vi "Stage 3.6 Placing GUI into subVIs.vi"() -> ()   [LabVIEW 2020]
panel:
  out "Process Error":errorcluster
  out "error out":errorcluster
  out "error out Hardware":errorcluster
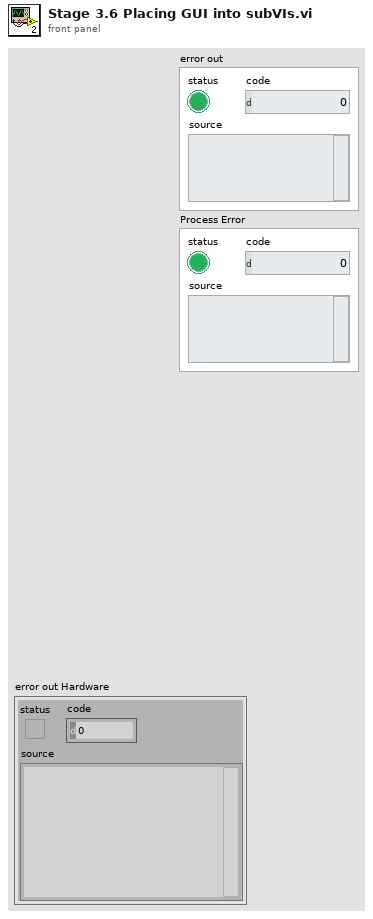
[diagram p1: front panel]
types:
  T1 = typedef "HRM-init_cluster.ctl" = cluster{"User events":T2}
  T2 = typedef "HRM-User_events.ctl" = cluster{"Signal to remove":refnum<user-event>, "Sample size":refnum<user-event>, "Filtered wf":refnum<user-event>, "Unfiltered wf":refnum<user-event>, "Raw wf":refnum<user-event>, "Pulse":refnum<user-event>, "stop":refnum<user-event>}
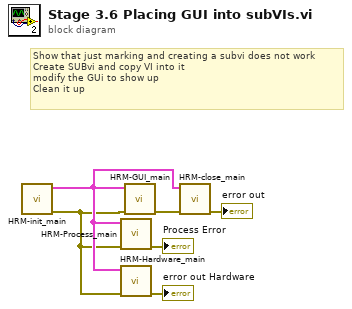
[diagram p0: block diagram]
diagram:
  # "Show that just marking and creating a subvi does not work\nCreate SUBvi and copy VI into it\nmodify the GUi to show up\nClean it up"
  n1 = call "HRM-init_main.vi"() -> ("error out"=w1:errorcluster, "Init cluster"=w3:T1)  [unwired: 10 in]
  n2 = call "HRM-Process_main.vi"("error in (no error)"=w1, "Init cluster"=w3) -> ("error out"=→"Process Error":errorcluster)  [unwired: 9 in]
  n3 = call "HRM-Hardware_main.vi"("error in (no error)"=w1, "Init cluster"=w3) -> ("error out"=→"error out Hardware":errorcluster)  [unwired: 9 in]
  n4 = call "HRM-GUI_main.vi"("error in (no error)"=w1, "Init cluster"=w3) -> ("error out"=w2:errorcluster)  [unwired: 9 in]
  n5 = call "HRM-close_main.vi"("error in (no error)"=w2, "Init cluster"=w3) -> ("error out"=→"error out":errorcluster)  [unwired: 9 in]
